vi "3.labtask3 (1).vi"() -> ()   [LabVIEW 2022 SP3]
panel:
  out "Waveform Chart":dynamicdata(graph)
  out "Total execution time (s)":u32
  out "Sampling period (ms)":dbl
  out "Total number of samples":dbl
  in  "Sampling rate (Hz)":dbl
  in  "Total duration (s)":dbl
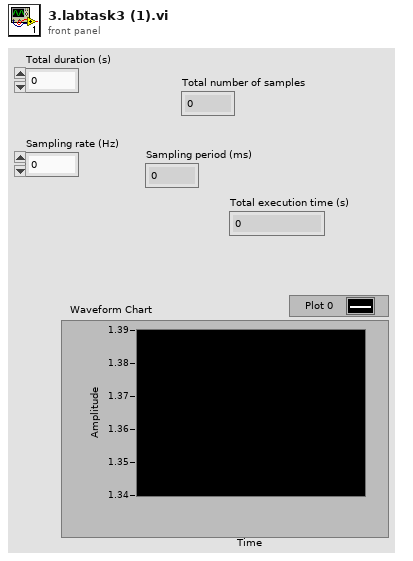
[diagram p1: front panel]
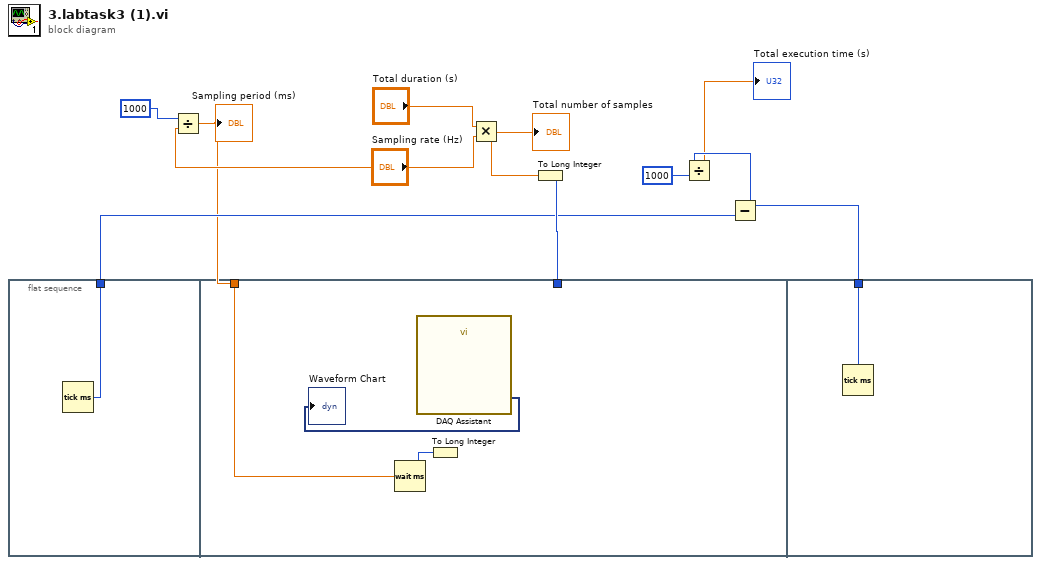
[diagram p0: block diagram]
diagram:
  n1 = flat-sequence {
    tunnel: [w12] -> w2
    tunnel: w7 -> [_]
    tunnel: w1 -> [w14]
    tunnel: [w16] -> w3
    frame #0 {
      n2 = Tick Count (ms)() -> (millisecond timer value=w12:u32)
    }
    frame #1 {
      n3 = Wait (ms)(milliseconds to wait=w14) -> (millisecond timer value=w13:u32)
      n4 = call "DAQ Assistant"() -> ("data"=→"Waveform Chart":dynamicdata)  [unwired: 17 in, 2 out]
      n5 = To Long Integer(number=w13) -> ()  [unwired: 1 out]
    }
    frame #2 {
      n6 = Tick Count (ms)() -> (millisecond timer value=w16:u32)
    }
  }
  n7 = Divide(x=1000, y="Sampling rate (Hz)") -> (x/y=w1:dbl)
  "Sampling period (ms)" <- w1
  n8 = Multiply(x="Total duration (s)", y="Sampling rate (Hz)") -> (x*y=w11:dbl)
  "Total number of samples" <- w11
  n9 = To Long Integer(number=w11) -> (32bit integer=w7:i32)
  n10 = Subtract(x=w3, y=w2) -> (x-y=w6:u32)
  n11 = Divide(x=w6, y=u32 1000) -> (x/y=→"Total execution time (s)":dbl)
